vi "ReportExpress_Mutation.vi"(0 "Diagram":refnum<vi>, 5 "ObjRef":refnum<vi>, 6 "Kind":string="SubVI", 7 "Information":string="<Not A Path>") -> (3 "Replace?":bool)   [LabVIEW 2020]
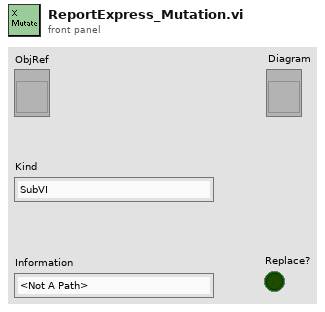
[diagram p1: front panel]
types:
  T1 = typedef "LVPositionTypeDef.ctl" = cluster{"Left":i32, "Top":i32}
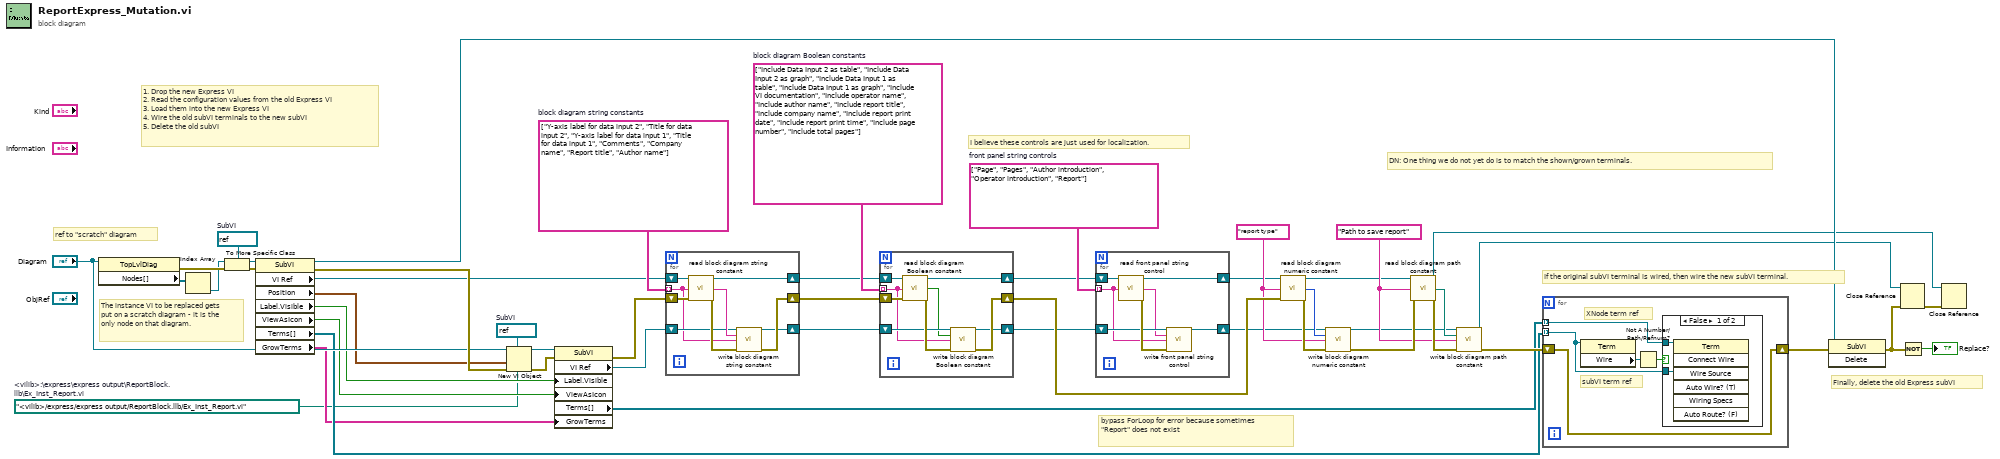
[diagram p0: block diagram]
diagram:
  w10 = string[] ["Page", "Pages", "Author introduction", "Operator introduction", "Report"]  # front panel string controls
  w14 = "Path to save report"
  w15 = "report type"
  w20 = string[] ["Y-axis label for data input 2", "Title for data input 2", "Y-axis label for data input 1", "Title for data input 1", "Comments", "Company name", "Report title", "Author name"]  # block diagram string constants
  w21 = string[] ["Include Data Input 2 as table", "Include Data Input 2 as graph", "Include Data Input 1 as table", "Include Data Input 1 as graph", "Include VI documentation", "Include operator name", "Include author name", "Include report title", "Include company name", "Include report print date", "Include report print time", "Include page number", "Include total pages"]  # block diagram Boolean constants
  w23 = path "<vilib>/express/express output/ReportBlock.llb/Ex_Inst_Report.vi"  # <vilib>:\express\express output\ReportBlock.llb\Ex_Inst_Report.vi
  w24 = refnum<vi> refnum  # SubVI
  w35 = refnum<vi> refnum  # SubVI
  # "bypass ForLoop for error because sometimes \"Report\" does not exist"
  # "DN: One thing we do not yet do is to match the shown/grown terminals."
  # "I believe these controls are just used for localization."
  # "Finally, delete the old Express subVI"
  # "If the original subVI terminal is wired, then wire the new subVI terminal."
  # "1. Drop the new Express VI\n2. Read the configuration values from the old Express VI\n3. Load them into the new Express VI\n4. Wire the old subVI terminals to the new subVI\n5. Delete the old subVI"
  # "The instance VI to be replaced gets put on a scratch diagram - it is the only node on that diagram."
  # "ref to \"scratch\" diagram"
  n1 = property class="TopLvlDiag"(reference="Diagram") -> (error out=w49:errorcluster, "Nodes[]"=w34:refnum<vi>[])  [unwired: 1 in, 1 out]
  n2 = Index Array(array=w34) -> (element=w33:refnum<vi>)  [unwired: 1 in]
  n3 = To More Specific Class(target class=w35, reference=w33, error in=w49) -> (specific class reference=w32:refnum<vi>, error out=w48:errorcluster)
  n4 = property class="SubVI"(reference=w32, error in=w48) -> (reference out=w28:refnum<vi>, error out=w36:errorcluster, "VI Ref"=w1:refnum<vi>, "Position"=w25:T1, "Label.Visible"=w26:bool, "ViewAsIcon"=w30:bool, "Terms[]"=w29:refnum<vi>[], "GrowTerms"=w27:string[])
  n5 = New VI Object(vi object class=w24, owner refnum="Diagram", position/next to=w25, 6:w23, 8:w36) -> (object refnum=w22:refnum<vi>, 0:w47:errorcluster)  [unwired: 3 in]
  n6 = property class="SubVI"(reference=w22, error in=w47, "Label.Visible"=w26, "ViewAsIcon"=w30, "GrowTerms"=w27) -> (error out=w43:errorcluster, "VI Ref"=w19:refnum<vi>, "Terms[]"=w5:refnum<vi>[])  [unwired: 1 out]
  n7 = for {
    shift-right: [w53] -> w18
    shift-left: w1 -> [w54]
    shift-right: [w51] -> w17
    shift-left: w19 -> [w52]
    shift-right: [w56] -> w42
    shift-left: w43 -> [w58]
    tunnel: w20 -> [w50] mode=indexing
    n8 = call <vilib>:"read block diagram string constant.vi"("VI Ref"=w54, "constant label"=w50, "error in"=w58) -> ("dup VI Ref"=w53:refnum<vi>, "constant string"=w55:string, "error out"=w57:errorcluster)  [unwired: 10 in]
    n9 = call <vilib>:"write block diagram string constant.vi"("VI Ref"=w52, "constant string"=w55, "constant label"=w50, "error in"=w57) -> ("dup VI Ref"=w51:refnum<vi>, "error out"=w56:errorcluster)  [unwired: 10 in]
  }
  n10 = for {
    shift-right: [w63] -> w9
    shift-left: w18 -> [w64]
    shift-right: [w61] -> w7
    shift-left: w17 -> [w62]
    shift-right: [w65] -> w37
    shift-left: w42 -> [w67]
    tunnel: w21 -> [w60] mode=indexing
    n11 = call <vilib>:"read block diagram Boolean constant.vi"("VI Ref"=w64, "constant label"=w60, "error in"=w67) -> ("dup VI Ref"=w63:refnum<vi>, "constant value"=w59:bool, "error out"=w66:errorcluster)  [unwired: 10 in]
    n12 = call <vilib>:"write block diagram Boolean constant.vi"("VI Ref"=w62, "constant Boolean"=w59, "constant label"=w60, "error in"=w66) -> ("dup VI Ref"=w61:refnum<vi>, "error out"=w65:errorcluster)  [unwired: 10 in]
  }
  n13 = for {
    shift-right: [w72] -> w8
    shift-left: w9 -> [w73]
    shift-right: [w70] -> w6
    shift-left: w7 -> [w71]
    tunnel: w10 -> [w69] mode=indexing
    n14 = call <vilib>:"read front panel string control.vi"("VI Ref"=w73, "control label"=w69) -> ("dup VI Ref"=w72:refnum<vi>, "string value"=w68:string, "error out"=w74:errorcluster)  [unwired: 11 in]
    n15 = call <vilib>:"write front panel string control.vi"("VI Ref"=w71, "string"=w68, "control label"=w69, "error in"=w74) -> ("dup VI Ref"=w70:refnum<vi>)  [unwired: 10 in, 1 out]
  }
  n16 = call <vilib>:"read block diagram numeric constant.vi"("VI Ref"=w8, "constant label"=w15, "error in"=w37) -> ("dup VI Ref"=w12:refnum<vi>, "constant value"=w16:i32, "error out"=w39:errorcluster)  [unwired: 10 in]
  n17 = call <vilib>:"write block diagram numeric constant.vi"("VI Ref"=w6, "constant numeric"=w16, "constant label"=w15, "error in"=w39) -> ("dup VI Ref"=w11:refnum<vi>, "error out"=w38:errorcluster)  [unwired: 10 in]
  n18 = call <vilib>:"read block diagram path constant.vi"("VI Ref"=w12, "constant label"=w14, "error in"=w38) -> ("dup VI Ref"=w3:refnum<vi>, "constant value"=w13:path, "error out"=w45:errorcluster)  [unwired: 10 in]
  n19 = call <vilib>:"write block diagram path constant.vi"("VI Ref"=w11, "constant path"=w13, "constant label"=w14, "error in"=w45) -> ("dup VI Ref"=w4:refnum<vi>, "error out"=w41:errorcluster)  [unwired: 10 in]
  n20 = for {
    tunnel: w29 -> [w75] mode=indexing
    tunnel: w5 -> [w76] mode=indexing
    shift-right: [w79] -> w46
    shift-left: w41 -> [w79]
    # "XNode term ref"
    # "subVI term ref"
    n21 = property class="Term"(reference=w75) -> ("Wire"=w78:refnum<vi>)  [unwired: 1 in, 2 out]
    n22 = Not A Number/Path/Refnum?(number/path/refnum=w78) -> (NaN/Path/Refnum?=w77:bool)
    n23 = case shown="False" w77 {
      tunnel: w75 -> [w81 _]
      tunnel: w76 -> [w80 _]
      frame False {
        n24 = invoke class="Term" method="Connect Wire"(reference=w80, "Wire Source"=w81) -> ()  [unwired: 5 in, 7 out]
      }
      frame True {
      }
    }
  }
  n25 = invoke class="SubVI" method="Delete"(reference=w28, error in=w46) -> (error out=w40:errorcluster)  [unwired: 1 in, 2 out]
  n26 = Close Reference(reference=w4, error in (no error)=w40) -> (error out=w44:errorcluster)
  n27 = Not(x=w40) -> (.not. x?=→"Replace?":bool)
  n28 = Close Reference(reference=w3, error in (no error)=w44) -> ()  [unwired: 1 out]
